vi "Symmetrical Components.vi"(8 "error in (no error)":errorcluster, 11 "3-phase phasors":cdb[](array[numeric])) -> (0 "error out":errorcluster, 1 "zero sequence":cdb, 2 "negative sequence":cdb, 3 "positive sequence":cdb)   [LabVIEW 2021]
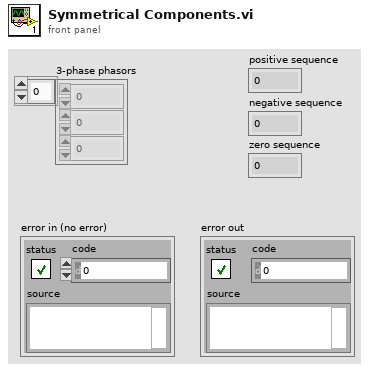
[diagram p1: front panel]
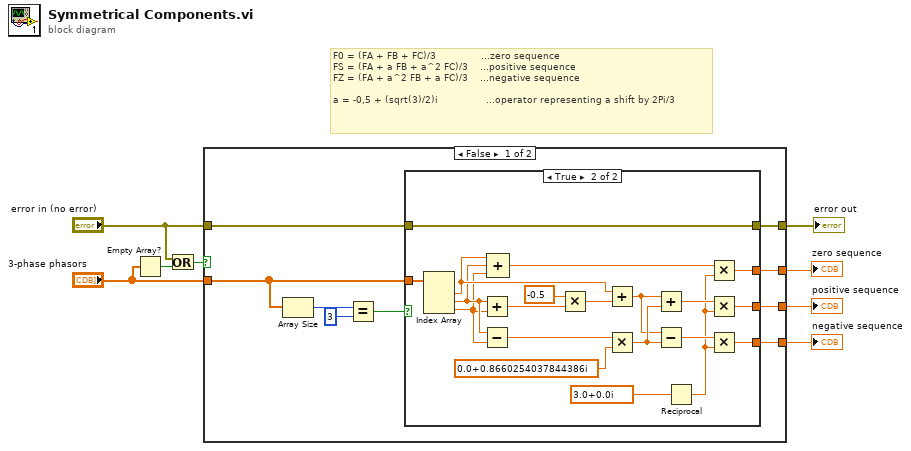
[diagram p0: block diagram]
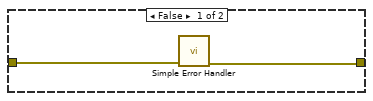
[diagram p2: hidden frame]
diagram:
  # "F0 = (FA + FB + FC)/3               ...zero sequence\nFS = (FA + a FB + a^2 FC)/3    ...positive sequence\nFZ = (FA + a^2 FB + a FC)/3    ...negative sequence\n\na = -0,5 + (sqrt(3)/2)i                ...operator representing a shift by 2Pi/3"
  n1 = Empty Array?(array="3-phase phasors") -> (empty?=w2:bool)
  n2 = Or(x="error in (no error)", y=w2) -> (x .or. y?=w4:bool)
  n3 = case shown="False" w4 {
    tunnel: "3-phase phasors" -> [w12 _]
    tunnel: [w17 _] -> w8
    tunnel: [w16 _] -> w7
    tunnel: [w15 _] -> w6
    tunnel: [w10 w40] -> w5
    tunnel: "error in (no error)" -> [w9 w40]
    frame False {
      n4 = Array Size(array=w12) -> (size(s)=w13:i32)
      n5 = Equal?(x=w13, y=3) -> (x = y?=w11:bool)
      n6 = case shown="True" w11 {
        tunnel: [_ w23] -> w17
        tunnel: [_ w22] -> w16
        tunnel: [_ w21] -> w15
        tunnel: w12 -> [_ w24]
        tunnel: [w18 w20] -> w10
        tunnel: w9 -> [w19 w20]
        frame False {
          n7 = call <vilib>:"Simple Error Handler.vi"("error in (no error)"=w19) -> ("error out"=w18:errorcluster)  [unwired: 4 in, 4 out]
        }
        frame True {
          n8 = Index Array(array=w24) -> (element #1=w27:cdb, element #2=w26:cdb, element #3=w25:cdb)  [unwired: 3 in]
          n9 = Add(x=w26, y=w25) -> (x+y=w31:cdb)
          n10 = Subtract(x=w26, y=w25) -> (x-y=w34:cdb)
          n11 = Compound Arithmetic op=ADD(w27, w26, w25) -> (w29:cdb)
          n12 = Multiply(x=-0.5 ("y"), y=w31) -> (x*y=w33:cdb)
          n13 = Add(x=w27, y=w33) -> (x+y=w36:cdb)
          n14 = Multiply(x=w34, y=cdb 0.0+0.8660254037844386i) -> (x*y=w37:cdb)
          n15 = Add(x=w36, y=w37) -> (x+y=w38:cdb)
          n16 = Subtract(x=w36, y=w37) -> (x-y=w39:cdb)
          n17 = Reciprocal(x=cdb 3.0+0.0i ("y")) -> (1/x=w30:cdb)
          n18 = Multiply(x=w29, y=w30) -> (x*y=w21:cdb)
          n19 = Multiply(x=w38, y=w30) -> (x*y=w23:cdb)
          n20 = Multiply(x=w39, y=w30) -> (x*y=w22:cdb)
        }
      }
    }
    frame True {
    }
  }
  "positive sequence" <- w8
  "negative sequence" <- w7
  "zero sequence" <- w6
  "error out" <- w5
